vi "OdorStim.vi"() -> ()   [LabVIEW 2012]
panel:
  in  "odor 2":bool
  in  "odor 1":bool
  in  "control stream":bool
  out "valves":bool[](array[boolean])
  in  "Post-Stim Time (s)":dbl=5.0
  in  "Stim Time (s)":dbl=2.0
  in  "Pre-Stim Time (s)":dbl=5.0
  out "Cycle#":i32=2
  in  "#Cycle":i32=2
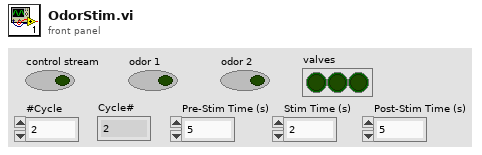
[diagram p1: front panel]
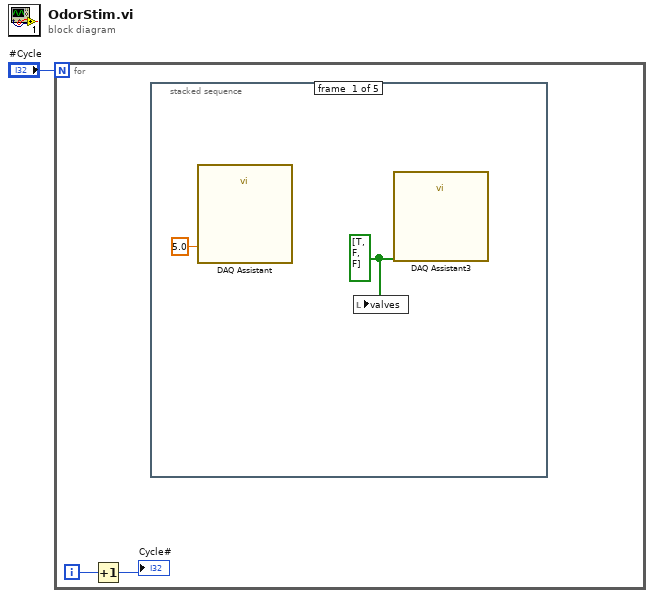
[diagram p0: block diagram]
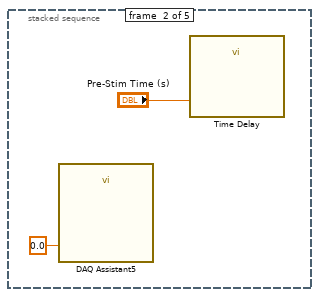
[diagram p2: hidden frame]
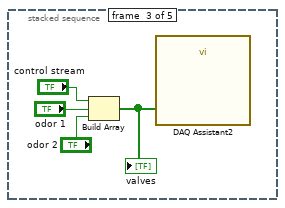
[diagram p3: hidden frame]
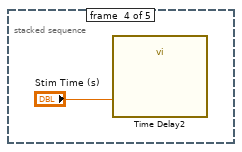
[diagram p4: hidden frame]
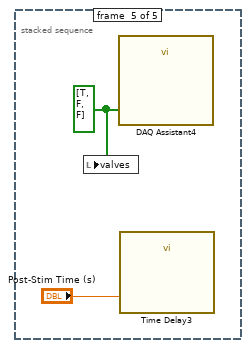
[diagram p5: hidden frame]
diagram:
  n1 = for {
    N: "#Cycle" -> [_]
    i -> [w3]
    n2 = Increment(x=w3) -> (x+1=→"Cycle#":i32)
    n3 = stacked-sequence {
      frame #0 {
        w4 = bool[] [TRUE, FALSE, FALSE] ("data")
        n4 = call "DAQ Assistant"("data"=5.0) -> ()  [unwired: 16 in, 3 out]
        n5 = local write "valves"(w4) -> ()
        n6 = call "DAQ Assistant3"("data"=w4) -> ()  [unwired: 17 in, 2 out]
      }
      frame #1 {
        n7 = call "DAQ Assistant5"("data"=0.0) -> ()  [unwired: 16 in, 3 out]
        n8 = call "Time Delay"("Delay Time (s)"="Pre-Stim Time (s)") -> ()  [unwired: 10 in, 1 out]
      }
      frame #2 {
        n9 = Build Array("control stream", "odor 1", "odor 2") -> (w8:bool[])
        "valves" <- w8
        n10 = call "DAQ Assistant2"("data"=w8) -> ()  [unwired: 17 in, 2 out]
      }
      frame #3 {
        n11 = call "Time Delay2"("Delay Time (s)"="Stim Time (s)") -> ()  [unwired: 10 in, 1 out]
      }
      frame #4 {
        w13 = bool[] [TRUE, FALSE, FALSE] ("data")
        n12 = local write "valves"(w13) -> ()
        n13 = call "DAQ Assistant4"("data"=w13) -> ()  [unwired: 17 in, 2 out]
        n14 = call "Time Delay3"("Delay Time (s)"="Post-Stim Time (s)") -> ()  [unwired: 10 in, 1 out]
      }
    }
  }
